vi "In Datei Loggen.vi"() -> (0 "error out":errorcluster)   [LabVIEW 2020, in "allgemeine Sub-VIs.lvlib"]
uses:
  allgemeine Sub-VIs.lvlib
  AK-Schnittstelle/AK-Schnittstelle.lvlib
  Stoerungen/Stoerungen.lvlib
  Funktionstasten/Funktionstasten.lvlib
  Schedule Modul/Schedule Modul.lvlib
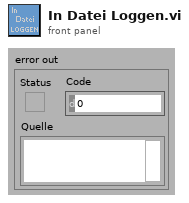
[diagram p1: front panel]
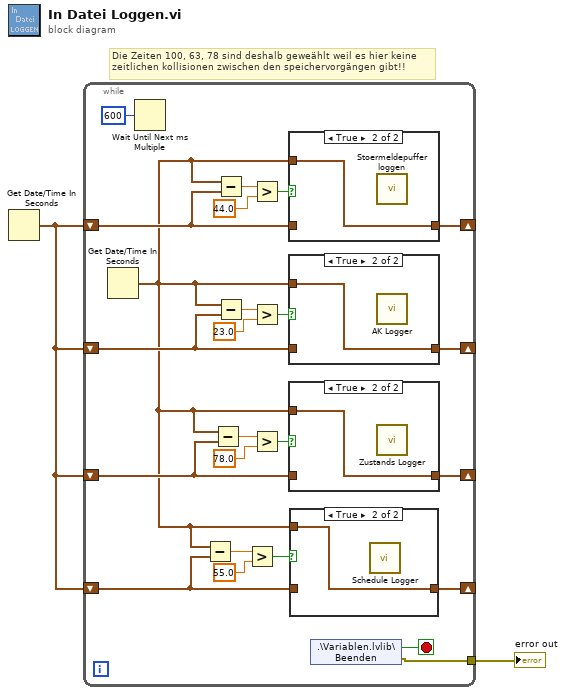
[diagram p0: block diagram]
diagram:
  # "Die Zeiten 100, 63, 78 sind deshalb geweählt weil es hier keine\nzeitlichen kollisionen zwischen den speichervorgängen gibt!!"
  n1 = Get Date/Time In Seconds() -> (seconds since 1Jan1904=w1:timestamp)
  n2 = while {
    shift-right: [w21] -> _
    shift-left: w1 -> [w22]
    shift-right: [w19] -> _
    shift-left: w1 -> [w13]
    shift-right: [w18] -> _
    shift-left: w1 -> [w11]
    tunnel: [w9] -> w2
    shift-right: [w8] -> _
    shift-left: w1 -> [w7]
    stop <- w20 stop-if-true
    n3 = Get Date/Time In Seconds() -> (seconds since 1Jan1904=w6:timestamp)
    n4 = Wait Until Next ms Multiple(millisecond multiple=u32 600 ("Vielfache von ms")) -> ()  [unwired: 1 out]
    n5 = Subtract(x=w6, y=w7) -> (x-y=w4:dbl)
    n6 = Subtract(x=w6, y=w11) -> (x-y=w16:dbl)
    n7 = Subtract(x=w6, y=w22) -> (x-y=w25:dbl)
    n8 = Subtract(x=w6, y=w13) -> (x-y=w17:dbl)
    n9 = Greater?(x=w4, y=55.0) -> (0:w5:bool)
    n10 = Greater?(x=w25, y=44.0) -> (0:w23:bool)
    n11 = Greater?(x=w17, y=23.0) -> (0:w14:bool)
    n12 = Greater?(x=w16, y=78.0) -> (0:w15:bool)
    n13 = case shown="True" w23 {
      tunnel: w6 -> [_ w34]
      tunnel: w22 -> [w33 _]
      tunnel: [w33 w34] -> w21
      frame False {
      }
      frame True {
        n14 = call "Stoermeldepuffer loggen.vi"() -> ()  [unwired: 12 in]
      }
    }
    n15 = case shown="True" w14 {
      tunnel: w6 -> [_ w32]
      tunnel: w13 -> [w31 _]
      tunnel: [w31 w32] -> w19
      frame False {
      }
      frame True {
        n16 = call "AK Logger.vi"() -> ()  [unwired: 12 in]
      }
    }
    n17 = case shown="True" w15 {
      tunnel: w6 -> [_ w30]
      tunnel: w11 -> [w29 _]
      tunnel: [w29 w30] -> w18
      frame False {
      }
      frame True {
        n18 = call "Zustands Logger.vi"() -> ()  [unwired: 12 in]
      }
    }
    n19 = case shown="True" w5 {
      tunnel: w7 -> [w27 _]
      tunnel: [w27 w28] -> w8
      tunnel: w6 -> [_ w28]
      frame False {
      }
      frame True {
        n20 = call "Schedule Logger.vi"() -> ()  [unwired: 12 in]
      }
    }
    n21 = shared-variable ".\\Variablen.lvlib\\Beenden"() -> (w20:bool, error out=w9:errorcluster)  [unwired: 1 in]
  }
  "error out" <- w2
